vi "Motion.ini.64postiions.vi"() -> ()   [LabVIEW 2017]
panel:
  out "error out":errorcluster
  in  "Cfg File path":path=path "C:/Users/Public/Documents/UCAR/APAR Board Test/SupportFiles/Motion64.ini"
  out "Cluster":T1={"64 postions"={"Antenna"=[{"X mm"=0.0, "Y mm"=0.0, "Z mm"=0.0, "T deg"=0.0}, {"X mm"=0.0, "Y mm"=0.0, "Z mm"=0.0, "T deg"=0.0}, {"X mm"=0.0, "Y mm"=0.0, "Z mm"=0.0, "T deg"=0.0}, {"X mm"=0.0, "Y mm"=0.0, "Z mm"=0.0, "T deg"=0.0}, {"X mm"=0.0, "Y mm"=0.0, "Z mm"=0.0, "T deg"=0.0}, {"X mm"=0.0, "Y mm"=0.0, "Z mm"=0.0, "T deg"=0.0}, {"X mm"=0.0, "Y mm"=0.0, "Z mm"=0.0, "T deg"=0.0}, {"X mm"=0.0, "Y mm"=0.0, "Z mm"=0.0, "T deg"=0.0}, {"X mm"=0.0, "Y mm"=0.0, "Z mm"=0.0, "T deg"=0.0}, {"X mm"=0.0, "Y mm"=0.0, "Z mm"=0.0, "T deg"=0.0}, {"X mm"=0.0, "Y mm"=0.0, "Z mm"=0.0, "T deg"=0.0}, {"X mm"=0.0, "Y mm"=0.0, "Z mm"=0.0, "T deg"=0.0}, {"X mm"=0.0, "Y mm"=0.0, "Z mm"=0.0, "T deg"=0.0}, {"X mm"=0.0, "Y mm"=0.0, "Z mm"=0.0, "T deg"=0.0}, {"X mm"=0.0, "Y mm"=0.0, "Z mm"=0.0, "T deg"=0.0}, {"X mm"=0.0, "Y mm"=0.0, "Z mm"=0.0, "T deg"=0.0}, {"X mm"=0.0, "Y mm"=0.0, "Z mm"=0.0, "T deg"=0.0}, {"X mm"=0.0, "Y mm"=0.0, "Z mm"=0.0, "T deg"=0.0}, {"X mm"=0.0, "Y mm"=0.0, "Z mm"=0.0, "T deg"=0.0}, {"X mm"=0.0, "Y mm"=0.0, "Z mm"=0.0, "T deg"=0.0}, {"X mm"=0.0, "Y mm"=0.0, "Z mm"=0.0, "T deg"=0.0}, {"X mm"=0.0, "Y mm"=0.0, "Z mm"=0.0, "T deg"=0.0}, {"X mm"=0.0, "Y mm"=0.0, "Z mm"=0.0, "T deg"=0.0}, {"X mm"=0.0, "Y mm"=0.0, "Z mm"=0.0, "T deg"=0.0}, {"X mm"=0.0, "Y mm"=0.0, "Z mm"=0.0, "T deg"=0.0}, {"X mm"=0.0, "Y mm"=0.0, "Z mm"=0.0, "T deg"=0.0}, {"X mm"=0.0, "Y mm"=0.0, "Z mm"=0.0, "T deg"=0.0}, {"X mm"=0.0, "Y mm"=0.0, "Z mm"=0.0, "T deg"=0.0}, {"X mm"=0.0, "Y mm"=0.0, "Z mm"=0.0, "T deg"=0.0}, {"X mm"=0.0, "Y mm"=0.0, "Z mm"=0.0, "T deg"=0.0}, {"X mm"=0.0, "Y mm"=0.0, "Z mm"=0.0, "T deg"=0.0}, {"X mm"=0.0, "Y mm"=0.0, "Z mm"=0.0, "T deg"=0.0}, {"X mm"=0.0, "Y mm"=0.0, "Z mm"=0.0, "T deg"=0.0}, {"X mm"=0.0, "Y mm"=0.0, "Z mm"=0.0, "T deg"=0.0}, {"X mm"=0.0, "Y mm"=0.0, "Z mm"=0.0, "T deg"=0.0}, {"X mm"=0.0, "Y mm"=0.0, "Z mm"=0.0, "T deg"=0.0}, {"X mm"=0.0, "Y mm"=0.0, "Z mm"=0.0, "T deg"=0.0}, {"X mm"=0.0, "Y mm"=0.0, "Z mm"=0.0, "T deg"=0.0}, {"X mm"=0.0, "Y mm"=0.0, "Z mm"=0.0, "T deg"=0.0}, {"X mm"=0.0, "Y mm"=0.0, "Z mm"=0.0, "T deg"=0.0}, {"X mm"=0.0, "Y mm"=0.0, "Z mm"=0.0, "T deg"=0.0}, {"X mm"=0.0, "Y mm"=0.0, "Z mm"=0.0, "T deg"=0.0}, {"X mm"=0.0, "Y mm"=0.0, "Z mm"=0.0, "T deg"=0.0}, {"X mm"=0.0, "Y mm"=0.0, "Z mm"=0.0, "T deg"=0.0}, {"X mm"=0.0, "Y mm"=0.0, "Z mm"=0.0, "T deg"=0.0}, {"X mm"=0.0, "Y mm"=0.0, "Z mm"=0.0, "T deg"=0.0}, {"X mm"=0.0, "Y mm"=0.0, "Z mm"=0.0, "T deg"=0.0}, {"X mm"=0.0, "Y mm"=0.0, "Z mm"=0.0, "T deg"=0.0}, {"X mm"=0.0, "Y mm"=0.0, "Z mm"=0.0, "T deg"=0.0}, {"X mm"=0.0, "Y mm"=0.0, "Z mm"=0.0, "T deg"=0.0}, {"X mm"=0.0, "Y mm"=0.0, "Z mm"=0.0, "T deg"=0.0}, {"X mm"=0.0, "Y mm"=0.0, "Z mm"=0.0, "T deg"=0.0}, {"X mm"=0.0, "Y mm"=0.0, "Z mm"=0.0, "T deg"=0.0}, {"X mm"=0.0, "Y mm"=0.0, "Z mm"=0.0, "T deg"=0.0}, {"X mm"=0.0, "Y mm"=0.0, "Z mm"=0.0, "T deg"=0.0}, {"X mm"=0.0, "Y mm"=0.0, "Z mm"=0.0, "T deg"=0.0}, {"X mm"=0.0, "Y mm"=0.0, "Z mm"=0.0, "T deg"=0.0}, {"X mm"=0.0, "Y mm"=0.0, "Z mm"=0.0, "T deg"=0.0}, {"X mm"=0.0, "Y mm"=0.0, "Z mm"=0.0, "T deg"=0.0}, {"X mm"=0.0, "Y mm"=0.0, "Z mm"=0.0, "T deg"=0.0}, {"X mm"=0.0, "Y mm"=0.0, "Z mm"=0.0, "T deg"=0.0}, {"X mm"=0.0, "Y mm"=0.0, "Z mm"=0.0, "T deg"=0.0}, {"X mm"=0.0, "Y mm"=0.0, "Z mm"=0.0, "T deg"=0.0}, {"X mm"=194.0, "Y mm"=194.0, "Z mm"=50.8, "T deg"=80.2}]}}
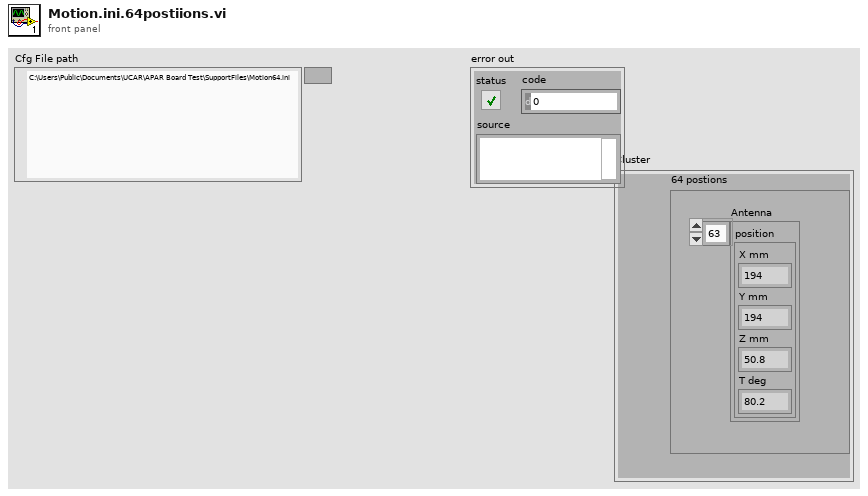
[diagram p1: front panel]
types:
  T1 = cluster{"64 postions":cluster{"Antenna":cluster{"X mm":dbl, "Y mm":dbl, "Z mm":dbl, "T deg":dbl}[]}}
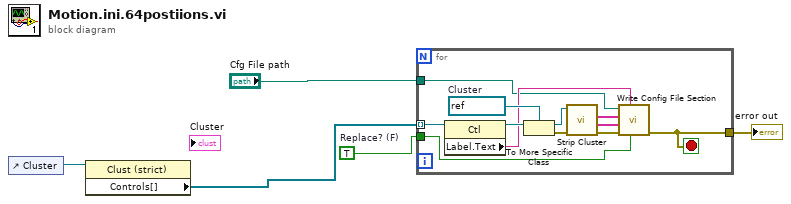
[diagram p0: block diagram]
diagram:
  w5 = TRUE  # Replace? (F)
  n1 = control-ref of="Cluster"() -> (w4:refnum<vi>)
  n2 = property class="Clust (strict)"(reference=w4) -> ("Controls[]"=w3:refnum<vi>[])  [unwired: 1 in, 2 out]
  n3 = for {
    tunnel: w3 -> [w10] mode=indexing
    tunnel: [w11] -> w1
    tunnel: w5 -> [w7]
    tunnel: "Cfg File path" -> [w6]
    stop <- w11 stop-if-true
    w17 = refnum<vi> refnum  # Cluster
    n4 = property class="Ctl"(reference=w10) -> (reference out=w9:refnum<vi>, "Label.Text"=w8:string)  [unwired: 1 in, 1 out]
    n5 = To More Specific Class(target class=w17, reference=w9) -> (specific class reference=w16:refnum<vi>, error out=w13:errorcluster)  [unwired: 1 in]
    n6 = call "Strip Cluster.vi"("error in (no error)"=w13, "Cluster Refnum"=w16) -> ("error out"=w12:errorcluster, "Values"=w14:string[], "Keys"=w15:string[])  [unwired: 6 in, 1 out]
    n7 = call "Write Config File Section.vi"("Replace? (F)"=w7, "Section"=w8, "error in"=w12, "Values"=w14, "Keys"=w15, "INI path"=w6) -> ("error out"=w11:errorcluster)  [unwired: 5 in]
  }
  "error out" <- w1
